vi "serial_terminal.vi"() -> ()   [LabVIEW 2010]
uses:
  <vilib>/Utility/semaphor.llb/Obtain Semaphore Reference.vi
  <vilib>/Instr/_visa.llb/VISA Configure Serial Port (Instr).vi
panel:
  in  "Convert special characters":bool=TRUE
  in  "Line ending":string="\r"
  in  "Stop communication":bool
  in  "COM port":refnum<visa-resource-name>
  in  "Baud rate":u32=38400
  in  "TX data":string
  out "Console log":string
  # "Configuration"
  # "Serial console"
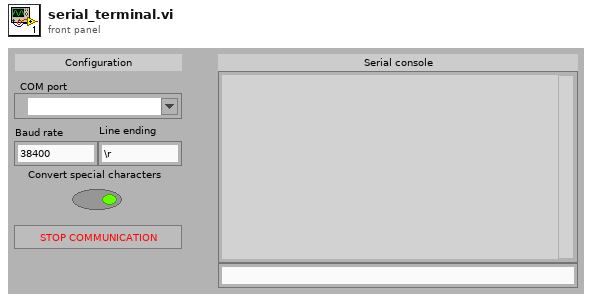
[diagram p1: front panel]
types:
  T1 = enum8{"Enabled", "Disabled", "Disabled and Grayed Out"}
  T2 = typedef "Semaphore RefNum" = refnum<k1>
  T3 = typedef "eventvkey.ctl" = enum16{"ASCII", "Enter", "Return", "Shift", "Ctrl", "Alt", "Cmd", "Opt", "Caps", "NumLock", "Clear", "Break", "Up", "Down", "Left", "Right", "Insert", "Delete", "Home", "End", "PageUp", "PageDown", "Escape", "Help", "Pause", "ScrollLock", "F1", "F2", "F3", "F4", "F5", "F6", "F7", "F8", "F9", "F10", "F11", "F12", "F13", "F14", "F15", "F16", "F17", "F18", "F19", "F20", "F21", "F22", "F23", "F24", "Play", "VolumeUp", "VolumeDown", "Mute", "Two Byte Char"}
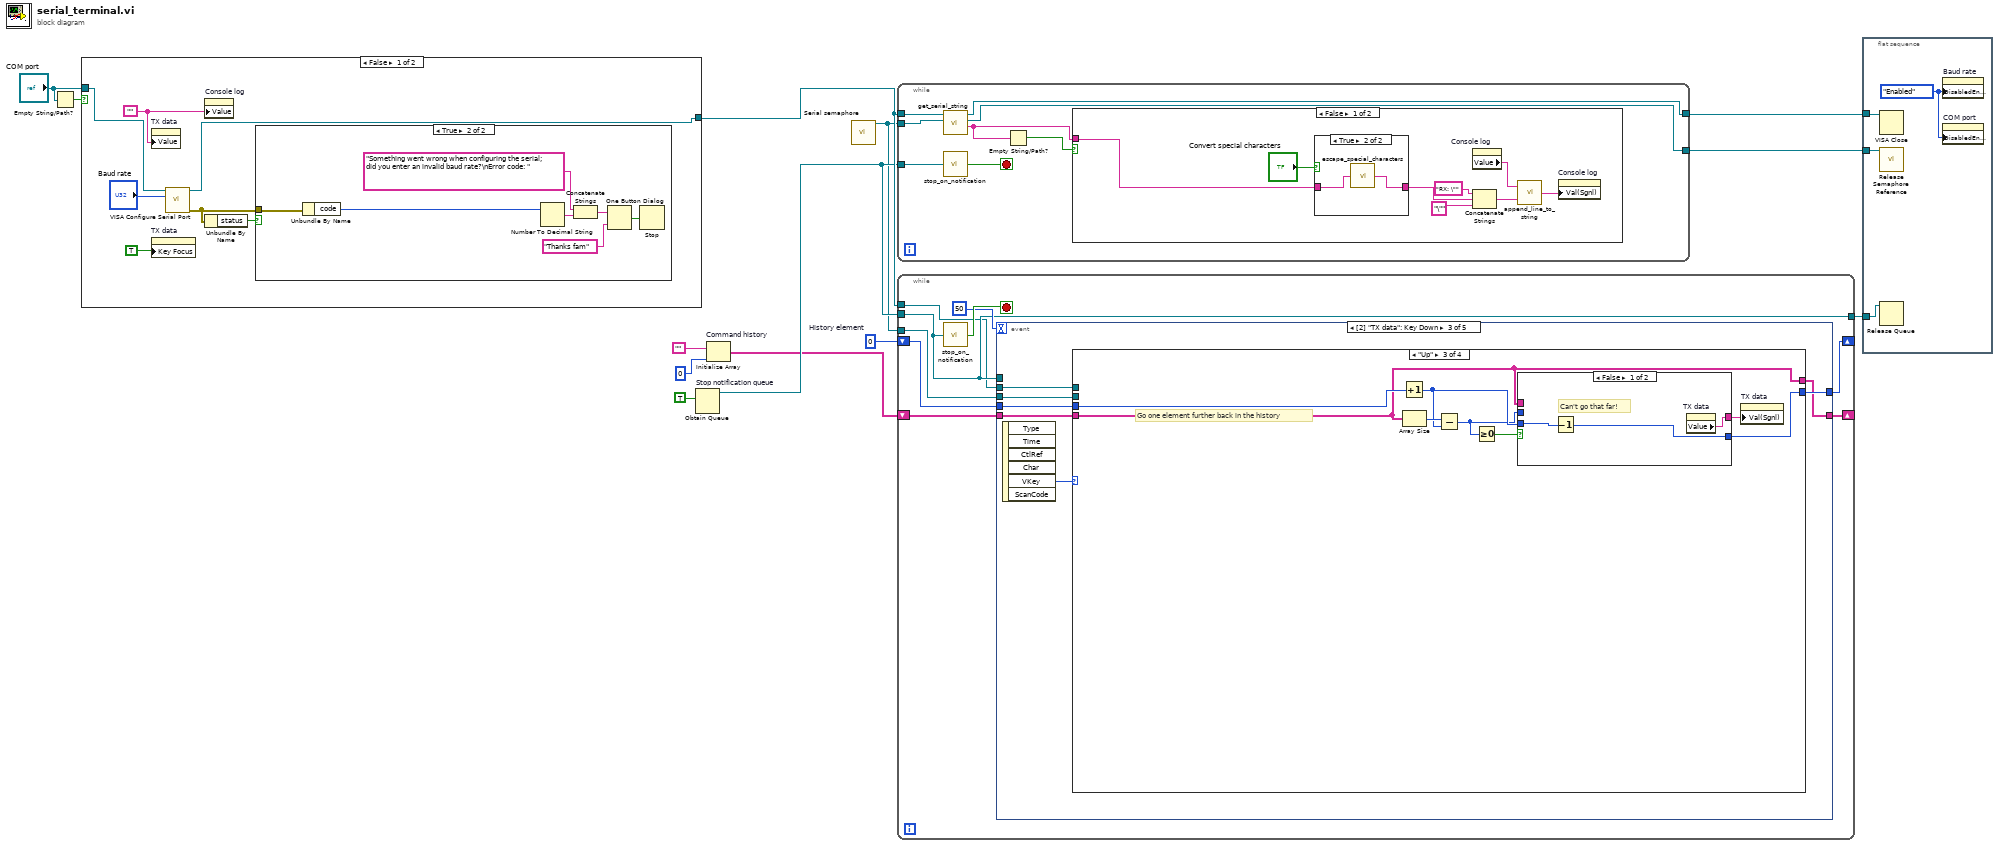
[diagram p0: block diagram]
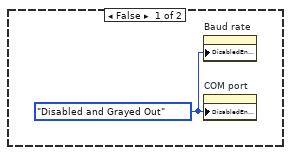
[diagram p2: hidden frame]
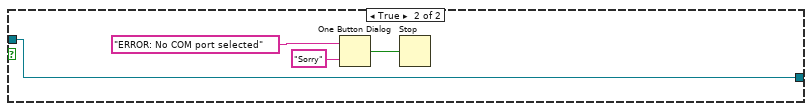
[diagram p3: hidden frame]
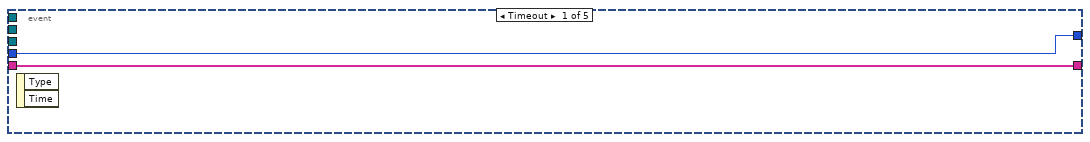
[diagram p4: hidden frame]
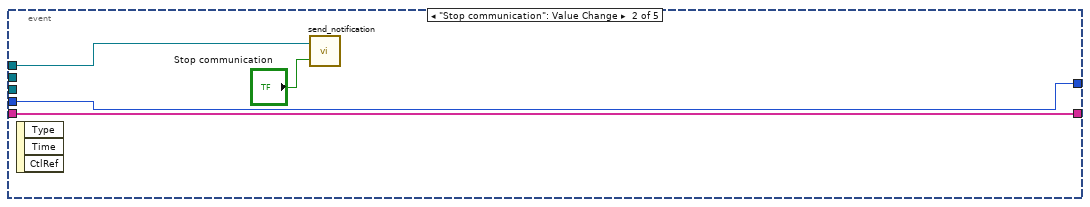
[diagram p5: hidden frame]
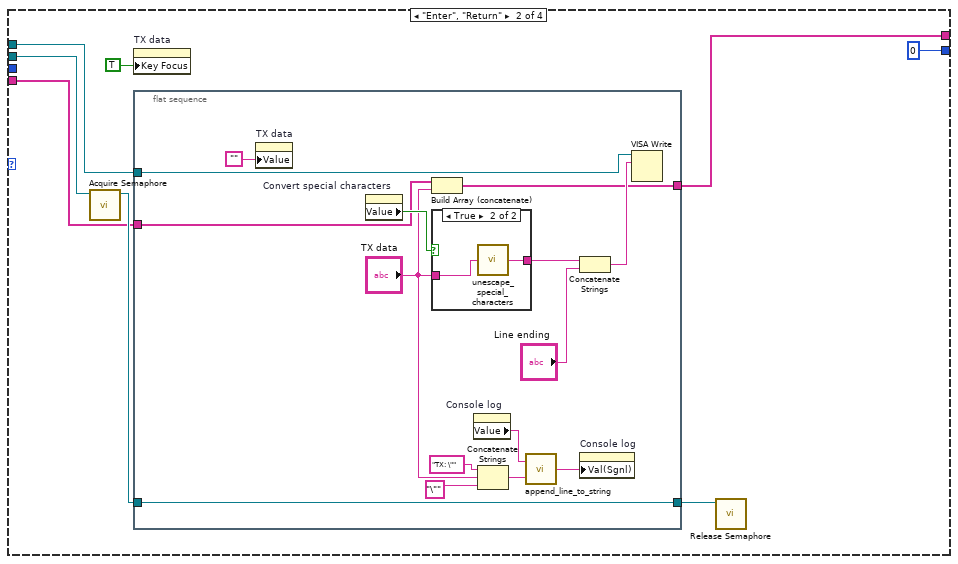
[diagram p7: hidden frame]
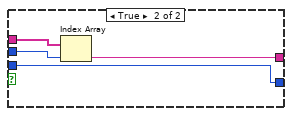
[diagram p9: hidden frame]
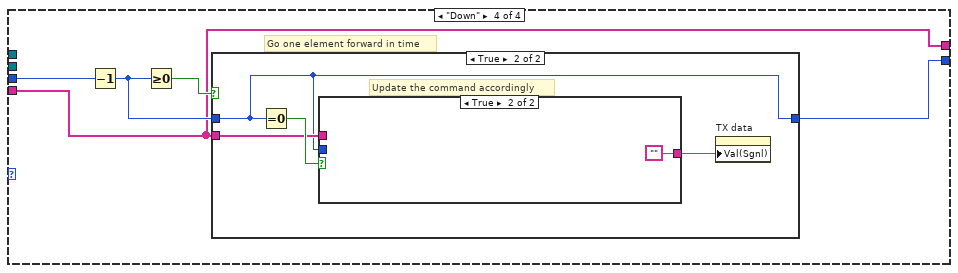
[diagram p10: hidden frame]
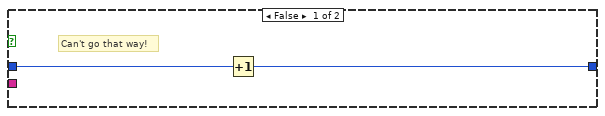
[diagram p11: hidden frame]
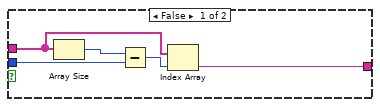
[diagram p12: hidden frame]
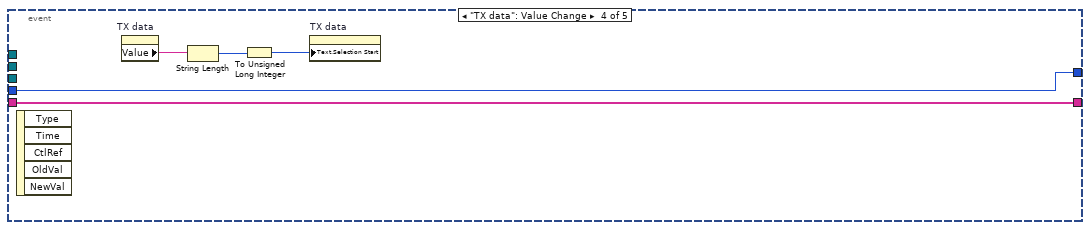
[diagram p13: hidden frame]
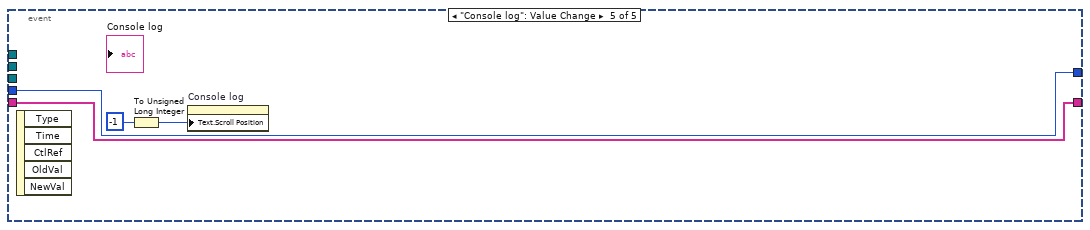
[diagram p14: hidden frame]
diagram:
  w1 = 0  # History element
  n1 = Empty String/Path?(string/path="COM port") -> (empty?=w9:bool)
  n2 = case shown="False" w9 {
    tunnel: [w19 w32] -> w8
    tunnel: "COM port" -> [w18 w32]
    frame False {
      w17 = ""
      n3 = property on="TX data" class="Str"("Value"=w17) -> ()  [unwired: 2 in, 2 out]
      n4 = property on="TX data" class="Str"("Key Focus"=TRUE) -> ()  [unwired: 2 in, 2 out]
      n5 = call-poly "VISA Configure Serial Port"("VISA resource name"=w18, "baud rate (9600)"="Baud rate") -> ("VISA resource name out"=w19:refnum<visa-resource-name>, "error out"=w14:errorcluster)  [unwired: 12 in]
      n6 = property on="Console log" class="Str"("Value"=w17) -> ()  [unwired: 2 in, 2 out]
      n7 = Unbundle By Name(w14) -> ("status"=w15:bool)
      n8 = case shown="True" w15 {
        tunnel: w14 -> [_ w27]
        frame False {
          w21 = T1."Disabled and Grayed Out" ("Disabled")
          n9 = property on="Baud rate" class="DigNum (strict)"("DisabledEnum"=w21) -> ()  [unwired: 2 in, 2 out]
          n10 = property on="COM port" class="VISAName"("DisabledEnum"=w21) -> ()  [unwired: 2 in, 2 out]
        }
        frame True {
          n11 = Unbundle By Name(w27) -> ("code"=w24:i32)
          n12 = Number To Decimal String(number=w24) -> (decimal integer string=w23:string)  [unwired: 1 in]
          n13 = Concatenate Strings("Something went wrong when configuring the serial; did you enter an invalid baud rate?\nError code: " ("message"), w23) -> (w26:string)
          n14 = One Button Dialog(message=w26, button name ("OK")="Thanks fam") -> (true=w22:bool)
          n15 = Stop(stop? (T)=w22) -> ()
        }
      }
    }
    frame True {
      n16 = One Button Dialog(message="ERROR: No COM port selected", button name ("OK")="Sorry") -> (true=w29:bool)
      n17 = Stop(stop? (T)=w29) -> ()
    }
  }
  n18 = Obtain Queue "Stop notification queue"(element data type=TRUE) -> (queue out=w6:refnum<queue>)  [unwired: 4 in, 2 out]
  n19 = Initialize Array "Command history"("", 0 ("dimension size")) -> (w2:string[])
  n20 = call "Serial semaphore"() -> ("semaphore"=w5:T2)  [unwired: 5 in, 2 out]
  n21 = while {
    tunnel: w8 -> [w37]
    tunnel: w6 -> [w39]
    tunnel: w5 -> [w38]
    tunnel: [w34] -> w11
    tunnel: [w33] -> w10
    stop <- w40 stop-if-true
    n22 = call "get_serial_string.vi"("Semaphore in"=w38, "VISA resource name in"=w37) -> ("Serial response"=w35:string, "Semaphore out"=w33:T2, "VISA resource name out"=w34:refnum<visa-resource-name>)  [unwired: 2 in, 1 out]
    n23 = call "stop_on_notification.vi"("Notofication queue"=w39) -> ("Should stop"=w40:bool)
    n24 = Empty String/Path?(string/path=w35) -> (empty?=w36:bool)
    n25 = case shown="False" w36 {
      tunnel: w35 -> [w42 _]
      frame False {
        n26 = case shown="True" "Convert special characters" {
          tunnel: w42 -> [w49 w51]
          tunnel: [w49 w50] -> w41
          frame False {
          }
          frame True {
            n27 = call "escape_special_characters.vi"("String in"=w51) -> ("String out"=w50:string)
          }
        }
        n28 = property on="Console log" class="Str"() -> ("Value"=w48:string)  [unwired: 2 in, 2 out]
        n29 = Concatenate Strings("RX: \"" ("string"), w41, "\"" ("string")) -> (w47:string)
        n30 = call "append_line_to_string.vi"("Line to add"=w47, "String in"=w48) -> ("String out"=w44:string)
        n31 = property on="Console log" class="Str"("Val(Sgnl)"=w44) -> ()  [unwired: 2 in, 2 out]
      }
      frame True {
      }
    }
  }
  n32 = while {
    tunnel: w6 -> [w58]
    tunnel: [w58] -> w12
    tunnel: w8 -> [w57]
    tunnel: w5 -> [w56]
    shift-right: [w53] -> _
    shift-left: w2 -> [w54]
    shift-right: [w52] -> _
    shift-left: w1 -> [w55]
    stop <- w60 stop-if-true
    n33 = call "stop_on_notification.vi"("Notofication queue"=w58) -> ("Should stop"=w60:bool)
    n34 = event shown="[2] \"TX data\": Key Down" {
      selector: _ -> [_ _ _ _ _]
      dyn-events: _ -> [_ _ _ _ _]
      timeout: 50 -> [_ _ _ _ _]
      tunnel: w58 -> [_ w65 _ _ _]
      tunnel: w57 -> [_ _ w73 _ _]
      tunnel: w56 -> [_ _ w72 _ _]
      tunnel: w55 -> [w61 w63 w70 w134 w139]
      tunnel: [w61 w63 w69 w134 w139] -> w52
      tunnel: w54 -> [w62 w64 w68 w135 w140]
      tunnel: [w62 w64 w67 w135 w140] -> w53
      event Timeout {
        n35 = event-data() -> ()  [unwired: 1 in, 2 out]
      }
      event "Stop communication": Value Change {
        n36 = event-data() -> ()  [unwired: 1 in, 3 out]
        n37 = call "send_notification.vi"("Notification"="Stop communication", "Notification queue in"=w65) -> ()  [unwired: 1 out]
      }
      event "TX data": Key Down {
        n38 = event-data() -> ("VKey"=w71:T3)  [unwired: 1 in, 5 out]
        n39 = case shown="\"Up\"" w71 {
          tunnel: w73 -> [_ w83 _ _]
          tunnel: w72 -> [_ w80 _ _]
          tunnel: w70 -> [w74 _ w109 w121]
          tunnel: [w74 0 w105 w118] -> w69
          tunnel: w68 -> [w75 w78 w103 w117]
          tunnel: [w75 w77 w103 w117] -> w67
          frame "ASCII", Default {
          }
          frame "Enter", "Return" {
            n40 = call <vilib>:"Acquire Semaphore.vi"("semaphore"=w80) -> ("semaphore out"=w82:T2)  [unwired: 4 in, 2 out]
            n41 = property on="TX data" class="Str"("Key Focus"=TRUE) -> ()  [unwired: 2 in, 2 out]
            n42 = flat-sequence {
              tunnel: w83 -> [w96]
              tunnel: w82 -> [w89]
              tunnel: [w89] -> w81
              tunnel: w78 -> [w86]
              tunnel: [w84] -> w77
              frame #0 {
                n43 = property on="TX data" class="Str"("Value"="") -> ()  [unwired: 2 in, 2 out]
                n44 = property on="Convert special characters" class="Bool (strict)"() -> ("Value"=w88:bool)  [unwired: 2 in, 2 out]
                n45 = Build Array (concatenate)(w86, "TX data") -> (w84:string[])
                n46 = case shown="True" w88 {
                  tunnel: "TX data" -> [w99 w101]
                  tunnel: [w99 w100] -> w87
                  frame False {
                  }
                  frame True {
                    n47 = call "unescape_special_characters.vi"("String in"=w101) -> ("String out"=w100:string)
                  }
                }
                n48 = property on="Console log" class="Str"() -> ("Value"=w94:string)  [unwired: 2 in, 2 out]
                n49 = Concatenate Strings("TX: \"" ("string"), "TX data", "\"" ("string")) -> (w93:string)
                n50 = call "append_line_to_string.vi"("Line to add"=w93, "String in"=w94) -> ("String out"=w95:string)
                n51 = Concatenate Strings(w87, "Line ending") -> (w97:string)
                n52 = property on="Console log" class="Str"("Val(Sgnl)"=w95) -> ()  [unwired: 2 in, 2 out]
                n53 = VISA Write(VISA resource name=w96, write buffer=w97) -> ()  [unwired: 1 in, 3 out]
              }
            }
            n54 = call <vilib>:"Release Semaphore.vi"("semaphore"=w81) -> ()  [unwired: 5 in, 2 out]
          }
          frame "Up" {
            # "Go one element further back in the history"
            n55 = Increment(x=w109) -> (x+1=w106:i32)
            n56 = Array Size(array=w103) -> (size(s)=w108:i32)
            n57 = Subtract(x=w108, y=w106) -> (x-y=w104:i32)
            n58 = Greater Or Equal To 0?(x=w104) -> (x >= 0?=w107:bool)
            n59 = case shown="False" w107 {
              tunnel: w106 -> [w112 w114]
              tunnel: [w111 w114] -> w105
              tunnel: w104 -> [_ w116]
              tunnel: w103 -> [_ w115]
              tunnel: [w110 w113] -> w102
              frame False {
                # "Can't go that far!"
                n60 = Decrement(x=w112) -> (x-1=w111:i32)
                n61 = property on="TX data" class="Str"() -> ("Value"=w110:string)  [unwired: 2 in, 2 out]
              }
              frame True {
                n62 = Index Array(array=w115, index=w116) -> (element=w113:string)
              }
            }
            n63 = property on="TX data" class="Str"("Val(Sgnl)"=w102) -> ()  [unwired: 2 in, 2 out]
          }
          frame "Down" {
            # "Go one element forward in time"
            n64 = Decrement(x=w121) -> (x-1=w119:i32)
            n65 = Greater Or Equal To 0?(x=w119) -> (x >= 0?=w120:bool)
            n66 = case shown="True" w120 {
              tunnel: w119 -> [w123 w125]
              tunnel: [w122 w125] -> w118
              tunnel: w117 -> [_ w126]
              frame False {
                # "Can't go that way!"
                n67 = Increment(x=w123) -> (x+1=w122:i32)
              }
              frame True {
                # "Update the command accordingly"
                n68 = Equal To 0?(x=w125) -> (x = 0?=w127:bool)
                n69 = case shown="True" w127 {
                  tunnel: [w128 ""] -> w124
                  tunnel: w126 -> [w132 _]
                  tunnel: w125 -> [w131 _]
                  frame False {
                    n70 = Array Size(array=w132) -> (size(s)=w130:i32)
                    n71 = Subtract(x=w130, y=w131) -> (x-y=w129:i32)
                    n72 = Index Array(array=w132, index=w129) -> (element=w128:string)
                  }
                  frame True {
                  }
                }
                n73 = property on="TX data" class="Str"("Val(Sgnl)"=w124) -> ()  [unwired: 2 in, 2 out]
              }
            }
          }
        }
      }
      event "TX data": Value Change {
        n74 = event-data() -> ()  [unwired: 1 in, 5 out]
        n75 = property on="TX data" class="Str"() -> ("Value"=w136:string)  [unwired: 2 in, 2 out]
        n76 = String Length(string=w136) -> (length=w137:i32)
        n77 = To Unsigned Long Integer(number=w137) -> (unsigned 32bit integer=w138:u32)
        n78 = property on="TX data" class="Str"("Text.Selection Start"=w138) -> ()  [unwired: 2 in, 2 out]
      }
      event "Console log": Value Change {
        n79 = event-data() -> ()  [unwired: 1 in, 5 out]
        n80 = To Unsigned Long Integer(number=-1) -> (unsigned 32bit integer=w142:u32)
        n81 = property on="Console log" class="Str"("Text.Scroll Position"=w142) -> ()  [unwired: 2 in, 2 out]
      }
    }
  }
  n82 = flat-sequence {
    tunnel: w12 -> [w146]
    tunnel: w11 -> [w145]
    tunnel: w10 -> [w144]
    frame #0 {
      w143 = T1."Enabled" ("Disabled")
      n83 = VISA Close(VISA resource name=w145) -> ()  [unwired: 1 in, 1 out]
      n84 = call <vilib>:"Release Semaphore Reference.vi"("semaphore"=w144) -> ()  [unwired: 9 in, 2 out]
      n85 = Release Queue(queue=w146) -> ()  [unwired: 2 in, 3 out]
      n86 = property on="Baud rate" class="DigNum (strict)"("DisabledEnum"=w143) -> ()  [unwired: 2 in, 2 out]
      n87 = property on="COM port" class="VISAName"("DisabledEnum"=w143) -> ()  [unwired: 2 in, 2 out]
    }
  }
